vi "GetType.vi"(8 "error in (no error)":errorcluster, 11 "Configure Arbitrary Waveform [ARB] Msg":refnum<class "Configure Arbitrary Waveform [ARB] Msg.lvclass">) -> (0 "error out":errorcluster, 2 "Data Sample":variant, 3 "Configure Arbitrary Waveform [ARB] Msg":refnum<class "Configure Arbitrary Waveform [ARB] Msg.lvclass">)   [LabVIEW 2015, in "CS++Fgen.lvlib" / "Configure Arbitrary Waveform [ARB] Msg.lvclass"]
doc: "This VI delivers a sample of the data type format the message expects."
uses:
  Configure Arbitrary Waveform [ARB] Msg.lvclass
  Configure Arbitrary Waveform [ARB] Msg.lvclass/Configure Arbitrary Waveform [ARB] Msg.ctl
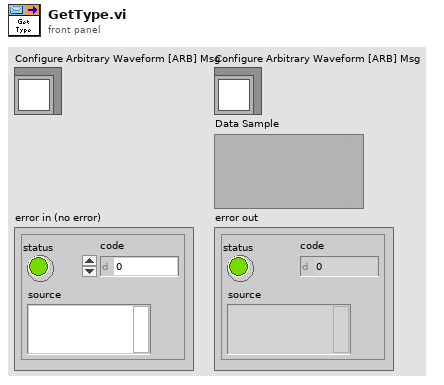
[diagram p1: front panel]
types:
  T1 = cluster{"channel name (\"CHANNEL1\")":string, "waveform handle (0)":i32, "gain (1.00)":dbl, "offset (0.00 V)":dbl[unit]}
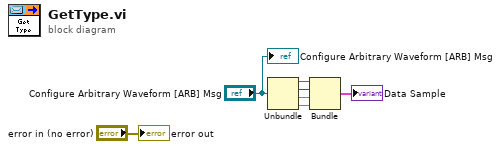
[diagram p0: block diagram]
diagram:
  n1 = Unbundle("Configure Arbitrary Waveform [ARB] Msg") -> (w4:string, w3:i32, w2:dbl, w1:dbl[unit])
  n2 = Bundle("channel name (\"CHANNEL1\")"=w4, "waveform handle (0)"=w3, "gain (1.00)"=w2, "offset (0.00 V)"=w1) -> (→"Data Sample":T1)  [unwired: 1 in]
  "error out" <- "error in (no error)"
  "Configure Arbitrary Waveform [ARB] Msg" <- "Configure Arbitrary Waveform [ARB] Msg"
